vi "Get stack data.vi"(8 "error in (no error)":errorcluster, 11 "Stack in":refnum<class "Stack.lvclass">) -> (0 "error out":errorcluster, 2 "Data cluster":T1={"type (proto/module)"="proto", " geometry"="full", "resolution"="LD", "baselayer"="BA_123", "toplayer"="SI_789", "bl_pos"="1", "tl_pos"="1", "put_pos"="1", "region"="1", "asstray"="1", "comptray"="1", "put"="1", "date"="2024-04-02", "timestart"="1:12:12.442", "timeend"="1:23:45.244", "operator"="cmuperson", "tape"="some", "glue"="some", "stack name"="some", "Adhesive type"="", "Comments"="", "Temperature"="", "Relative Humidity"=""}, 3 "Stack out":refnum<class "Stack.lvclass">)   [LabVIEW 2021, in "Stack.lvclass"]
uses:
  Stack.lvclass
  Stack.lvclass/Stack.ctl
panel:
  # "Debug Instructions\n#### The order of values in db_data_cols must match the order of values in Data cluster in Stack.lvclass: Get stack data.vi \n#### The variable names below correspond to postgres col name. LV does not neet to match the col numes but just the values. \n#### Right-click on the Data cluster on the front panel and click on 'reorder controls' to verify the order is correct in the code. \n#### The physical position of the fields is different from the actual position.\n\nIn Main VIs/python_db/postgres_tools.py, see functions 'assembly_data' and 'assembly_data_as_list'."
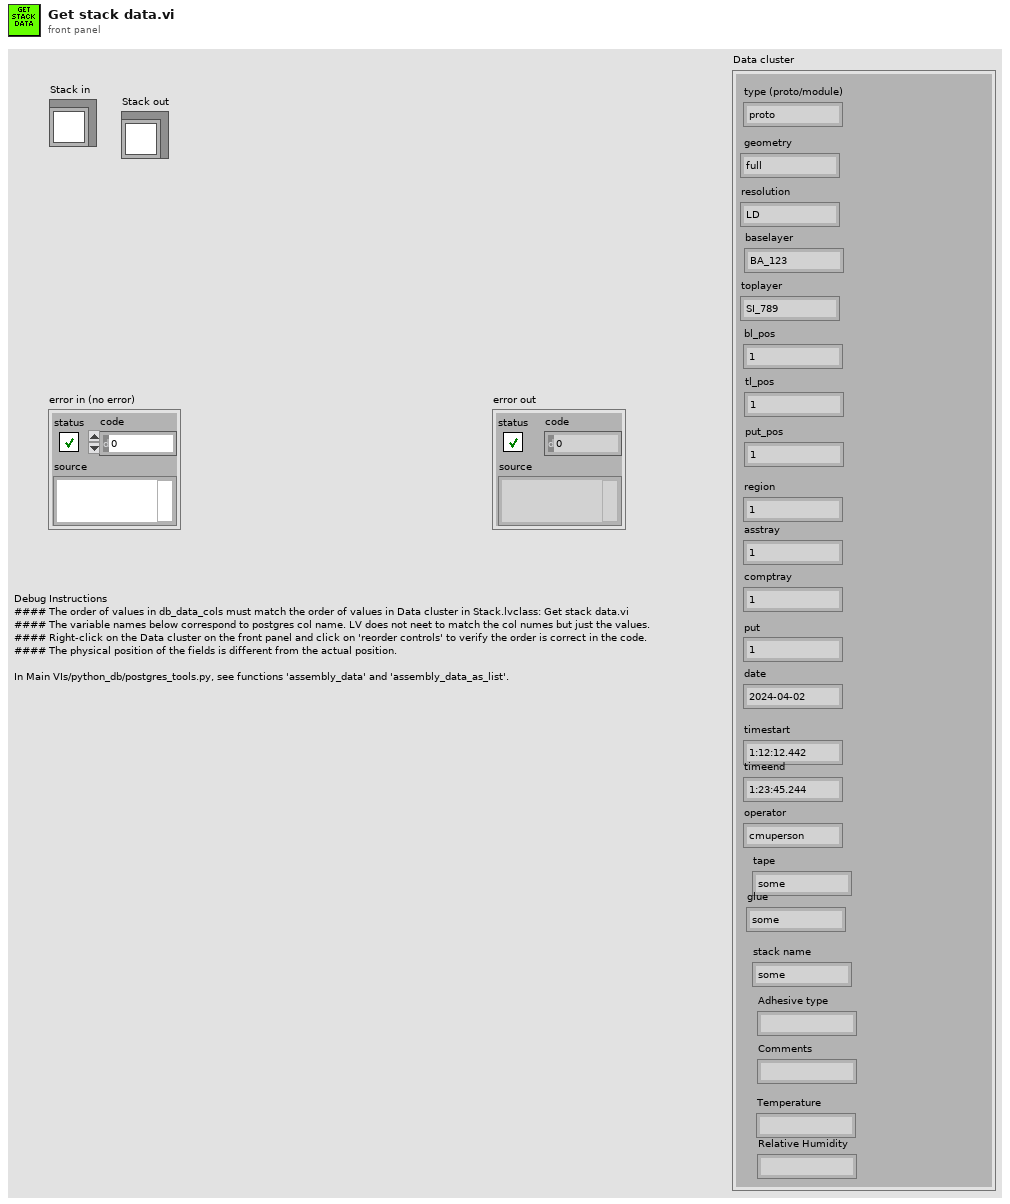
[diagram p1: front panel]
types:
  T1 = cluster{"type (proto/module)":string, " geometry":string, "resolution":string, "baselayer":string, "toplayer":string, "bl_pos":string, "tl_pos":string, "put_pos":string, "region":string, "asstray":string, "comptray":string, "put":string, "date":string, "timestart":string, "timeend":string, "operator":string, "tape":string, "glue":string, "stack name":string, "Adhesive type":string, "Comments":string, "Temperature":string, "Relative Humidity":string}
  T2 = cluster{"type":string, " geometry":string, "resolution":string, "baselayer":string, "toplayer":string, "bl_pos":string, "tl_pos":string, "put_pos":string, "region":string, "asstray":string, "comptray":string, "put":string, "date":string, "timestart":string, "timeend":string, "operator":string, "tape":string, "glue":string, "stack name":string, "Adhesive type":string, "Comments":string, "Temperature":string, "Relative Humidity":string}
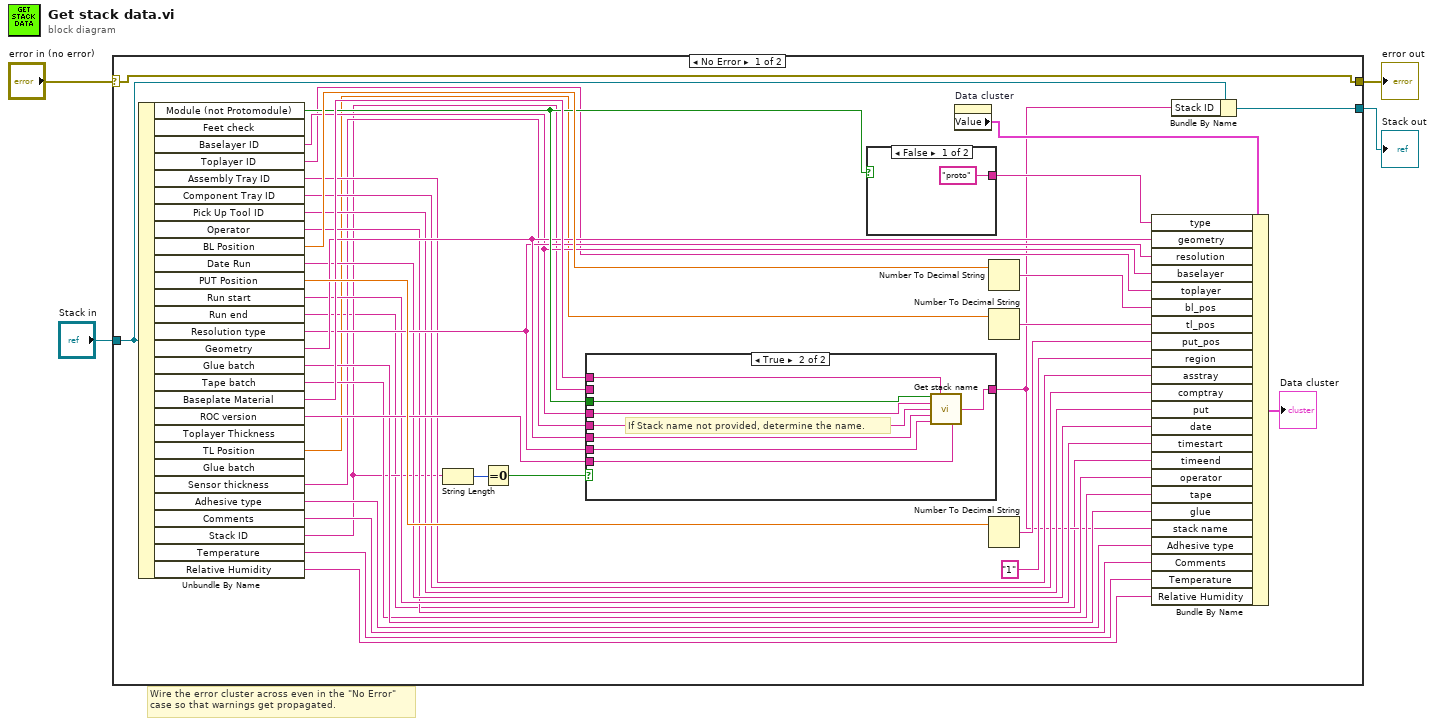
[diagram p0: block diagram]
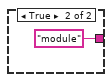
[diagram p3: hidden frame]
diagram:
  # "Wire the error cluster across even in the \"No Error\"\ncase so that warnings get propagated."
  n1 = case shown="No Error" "error in (no error)" {
    selector: "error in (no error)" -> [w42 w55]
    tunnel: [w42 w55] -> w3
    tunnel: [w8 w54] -> w1
    tunnel: "Stack in" -> [w7 w54]
    frame No Error {
      n2 = Unbundle By Name(w7) -> ("Module (not Protomodule)"=w38:bool, "Baselayer ID"=w31:string, "Toplayer ID"=w30:string, "Assembly Tray ID"=w29:string, "Component Tray ID"=w28:string, "Pick Up Tool ID"=w27:string, "Operator"=w24:string, "BL Position"=w41:dbl, "Date Run"=w26:string, "PUT Position"=w40:dbl, "Run start"=w25:string, "Run end"=w5:string, "Resolution type"=w32:string, "Geometry"=w33:string, "Glue batch"=w23:string, "Tape batch"=w22:string, "Baseplate Material"=w39:string, "ROC version"=w37:string, "TL Position"=w21:dbl, "Sensor thickness"=w16:string, "Adhesive type"=w15:string, "Comments"=w14:string, "Stack ID"=w11:string, "Temperature"=w10:string, "Relative Humidity"=w9:string)  [unwired: 3 out]
      n3 = String Length(string=w11) -> (length=w13:i32)
      n4 = Equal To 0?(x=w13) -> (x = 0?=w12:bool)
      n5 = case shown="True" w12 {
        tunnel: w39 -> [_ w51]
        tunnel: w38 -> [_ w50]
        tunnel: w37 -> [_ w49]
        tunnel: [w43 w48] -> w6
        tunnel: w33 -> [_ w47]
        tunnel: w32 -> [_ w46]
        tunnel: w31 -> [_ w45]
        tunnel: w16 -> [_ w44]
        tunnel: w11 -> [w43 _]
        frame False {
        }
        frame True {
          # "If Stack name not provided, determine the name."
          n6 = call "Get stack name.vi"("Module?"=w50, "Baseplate Type"=w51, "Protoname (baselayer)"=w45, "Sensor thickness"=w44, "Geometry"=w47, "Resolution"=w46, "Hexaboard ROC version"=w49) -> ("Stack name"=w48:string)  [unwired: 8 in]
        }
      }
      n7 = case shown="False" w38 {
        tunnel: ["proto" ("type") "module" ("type")] -> w34
        frame False {
        }
        frame True {
        }
      }
      n8 = property on="Data cluster" class="Clust (strict)"() -> ("Value"=w35:T2)  [unwired: 2 in, 2 out]
      n9 = Number To Decimal String(number=w41) -> (decimal integer string=w19:string)  [unwired: 1 in]
      n10 = Number To Decimal String(number=w21) -> (decimal integer string=w20:string)  [unwired: 1 in]
      n11 = Number To Decimal String(number=w40) -> (decimal integer string=w18:string)  [unwired: 1 in]
      n12 = Bundle By Name(cluster=w35, "type"=w34, "geometry"=w33, "resolution"=w32, "baselayer"=w31, "toplayer"=w30, "bl_pos"=w19, "tl_pos"=w20, "put_pos"=w18, "region"="1", "asstray"=w29, "comptray"=w28, "put"=w27, "date"=w26, "timestart"=w25, "timeend"=w5, "operator"=w24, "tape"=w22, "glue"=w23, "stack name"=w6, "Adhesive type"=w15, "Comments"=w14, "Temperature"=w10, "Relative Humidity"=w9) -> (→"Data cluster":T2)
      n13 = Bundle By Name(cluster=w7, "Stack ID"=w6) -> (w8:refnum<class "Stack.lvclass">)
    }
    frame Error {
    }
  }
  "error out" <- w3
  "Stack out" <- w1
